vi "Configure Auto Calibrate.vi"(8 "error in (no error)":errorcluster, 10 "Auto Calibrate (T: Enable)":bool=TRUE, 11 "VISA resource name":refnum<visa-resource-name>) -> (0 "error out":errorcluster, 3 "VISA resource name out":refnum<visa-resource-name>)   [LabVIEW 2014, in "Agilent U2000 Series.lvlib"]
doc: "Enables or disables auto calibrate.\n\nNote:\nThis VI is applicable for Agilent U2021/2XA and U2040 X-Series only."
uses:
  Agilent U2000 Series.lvlib
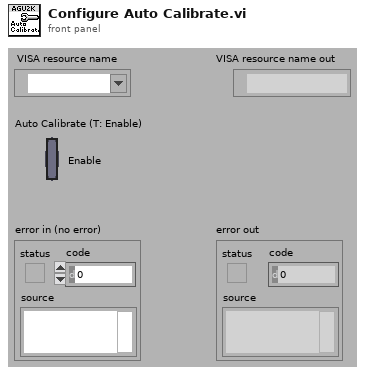
[diagram p1: front panel]
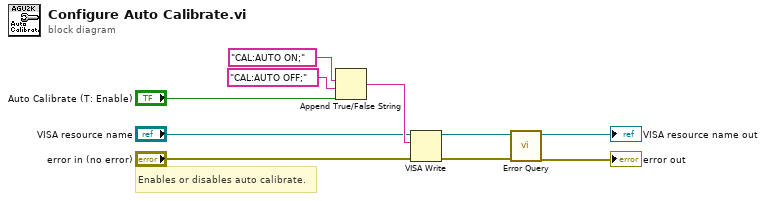
[diagram p0: block diagram]
diagram:
  # "Enables or disables auto calibrate."
  n1 = Append True/False String(1:"Auto Calibrate (T: Enable)", 2:"CAL:AUTO OFF;", 3:"CAL:AUTO ON;") -> (0:w7:string)  [unwired: 1 out]
  n2 = VISA Write(VISA resource name="VISA resource name", write buffer=w7, error in (no error)="error in (no error)") -> (VISA resource name out=w4:refnum<visa-resource-name>, error out=w3:errorcluster)  [unwired: 1 out]
  n3 = call "Error Query.vi"("error in (no error)"=w3, "VISA resource name"=w4) -> ("error out"=→"error out":errorcluster, "VISA resource name out"=→"VISA resource name out":refnum<visa-resource-name>)  [unwired: 8 out]
